vi "DestroyUserEvents.vi"(8 "error in (no error)":errorcluster, 11 "User Event in":refnum<class "User Event.lvclass">) -> (0 "error out":errorcluster, 3 "User Event out":refnum<class "User Event.lvclass">)   [LabVIEW 2016, in "User Event.lvclass"]
uses:
  User Event.lvclass
  User Event.lvclass/User Event.ctl
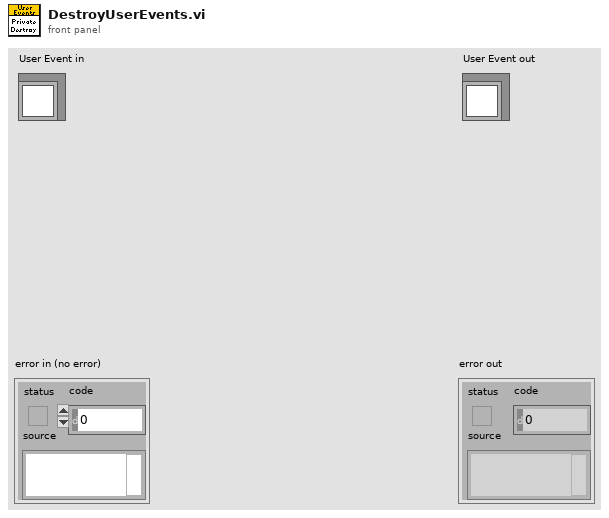
[diagram p1: front panel]
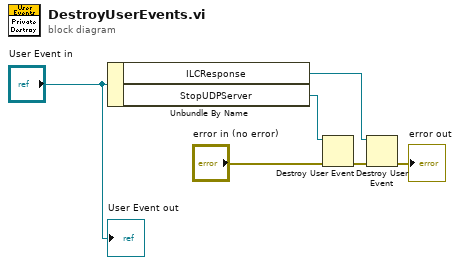
[diagram p0: block diagram]
diagram:
  n1 = Unbundle By Name("User Event in") -> ("ILCResponse"=w4:refnum<user-event>, "StopUDPServer"=w6:refnum<user-event>)
  n2 = Destroy User Event(user event=w6, error in="error in (no error)") -> (error out=w5:errorcluster)
  n3 = Destroy User Event(user event=w4, error in=w5) -> (error out=→"error out":errorcluster)
  "User Event out" <- "User Event in"
